vi "Error_and_Status_Unit_Test.vi"() -> ()   [LabVIEW 2017]
uses:
  Controls/Control Packets/ES_Param.ctl
  Controls/Packet/Packet.ctl
  Controls/Packet/Packet_Direction.ctl
  Controls/Packet/Packet_Type.ctl
  Controls/Packet/Packet_Priority.ctl
panel:
  out "ES Packet Out":T1
  out "ES Param Out":T5
  in  "Retry interval (ms)":u32
  in  "Number of tries":u32
  in  "baud rate":u32=9600
  in  "COM Port In":refnum<visa-resource-name>
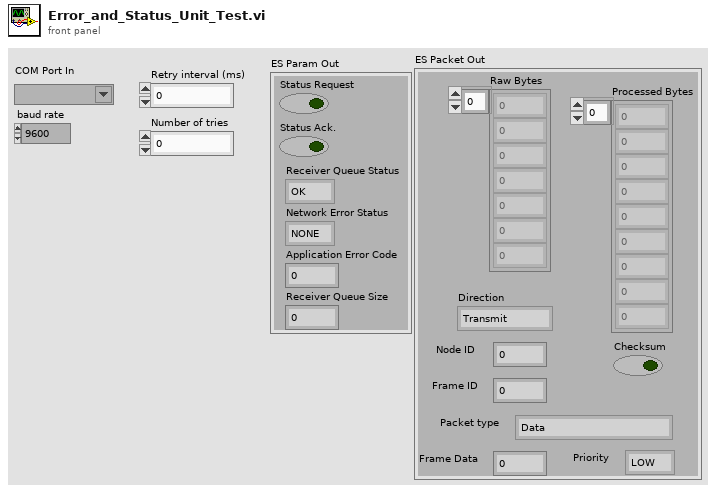
[diagram p1: front panel]
types:
  T1 = typedef "Packet.ctl" = cluster{"Raw Bytes":u8[], "Checksum":bool, "Direction":T2, "Processed Bytes":u8[], "Node ID":u8, "Packet type":T3, "Frame Data":u32, "Priority":T4, "Frame ID":u8}
  T2 = typedef "Packet_Direction.ctl" = enum16{"Transmit", "Receive", "Bidirectional"}
  T3 = typedef "Packet_Type.ctl" = enum16{"Data", "Connection Management", "Remote Request", "Error/Status"}
  T4 = typedef "Packet_Priority.ctl" = enum16{"LOW", "HIGH"}
  T5 = typedef "ES_Param.ctl" = cluster{"Status Request":bool, "Status Ack.":bool, "Receiver Queue Status":enum16{"OK", "EMPTY", "FULL"}, "Network Error Status":enum16{"NONE", "CONNECTION_ALREADY_OPEN", "CONNECTION_ALREADY_CLOSED", "INVALID_FRAME_REQUEST"}, "Application Error Code":u16, "Receiver Queue Size":i32}
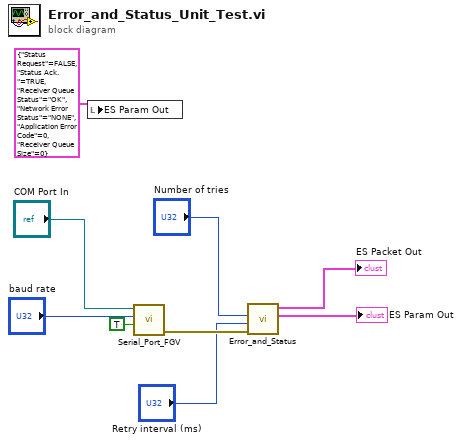
[diagram p0: block diagram]
diagram:
  n1 = local write "ES Param Out"(T5 {"Status Request"=FALSE, "Status Ack."=TRUE, "Receiver Queue Status"=enum."OK", "Network Error Status"=enum."NONE", "Application Error Code"=0, "Receiver Queue Size"=0} ("ES Param Out")) -> ()
  n2 = call "Serial_Port_FGV.vi"("Initialize ?"=TRUE, "baud rate"="baud rate", "COM Port In"="COM Port In") -> ("error out"=w6:errorcluster)  [unwired: 7 in, 1 out]
  n3 = call "Error_and_Status.vi"("error in (no error)"=w6, "Retry interval (ms)"="Retry interval (ms)", "Number of tries"="Number of tries") -> ("ES Param Out"=→"ES Param Out":T5, "ES Packet Out"=→"ES Packet Out":T1)  [unwired: 6 in, 1 out]
